vi "GuiPanelClose.vi"(8 "error in (no error)":errorcluster, 11 "CallerMessage in":refnum<class "CallerMessage.lvclass">) -> (0 "error out":errorcluster, 3 "CallerMessage out":refnum<class "CallerMessage.lvclass">)   [LabVIEW 2022 SP3, in "Gui.lvlib" / "CallerMessage.lvclass"]
uses:
  CallerMessage.lvclass
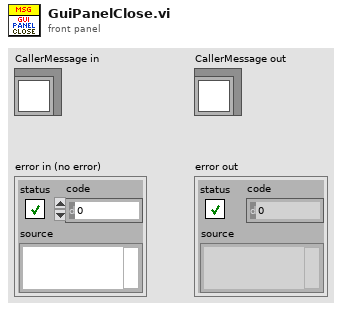
[diagram p1: front panel]
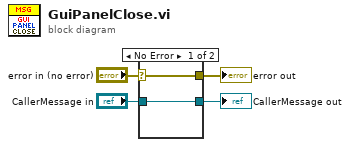
[diagram p0: block diagram]
diagram:
  n1 = case shown="No Error" "error in (no error)" {
    selector: "error in (no error)" -> [w5 w8]
    tunnel: [w5 w8] -> w3
    tunnel: [w6 w7] -> w1
    tunnel: "CallerMessage in" -> [w6 w7]
    frame No Error {
    }
    frame Error {
    }
  }
  "error out" <- w3
  "CallerMessage out" <- w1
